vi "Element to JSON.vi"(8 "error in (no error)":errorcluster, 10 "Element":refnum<class "Config Element.lvclass">, 11 "Config-JSON":refnum<class "Config-JSON.lvclass">) -> (0 "error out":errorcluster, 2 "JSON":string)   [LabVIEW 2020, in "CDM-Config.lvlib" / "Config-JSON.lvclass"]
uses:
  Config-JSON.lvclass
  Config Element/Config Element.lvclass
  C:/dev/lv20CE/relink/lv-cdm/CDM-Config/Config Storage/Config Storage.lvclass
  Config Storage/Config Storage.lvclass
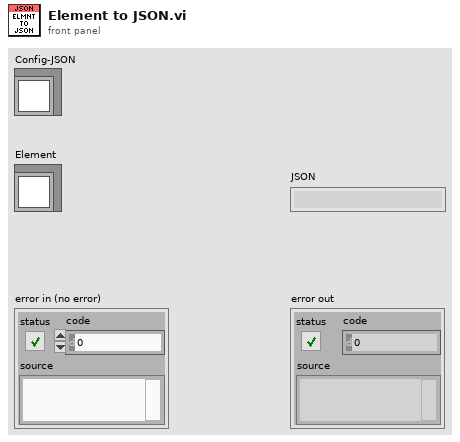
[diagram p1: front panel]
types:
  T1 = typedef "CDM-Config.lvlib/Value Type.ctl" = enum16{"String", "Number", "Bool", "Object", "Array"}
  T2 = typedef "CDM-Config.lvlib/Meta Data.ctl" = cluster{"Name":string, "Value":string}
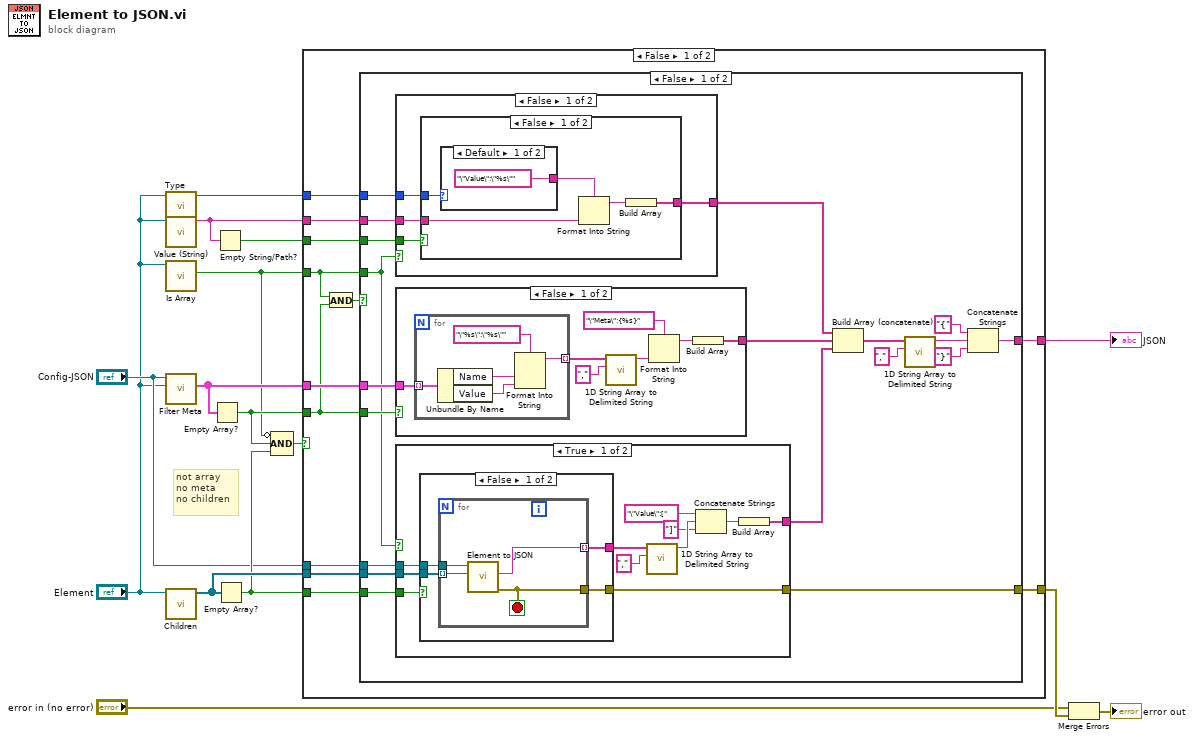
[diagram p0: block diagram]
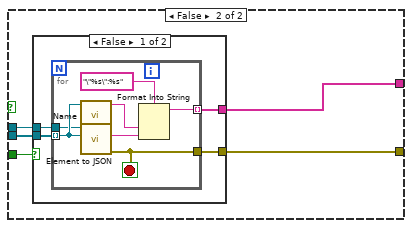
[diagram p3: hidden frame]
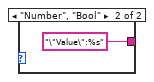
[diagram p5: hidden frame]
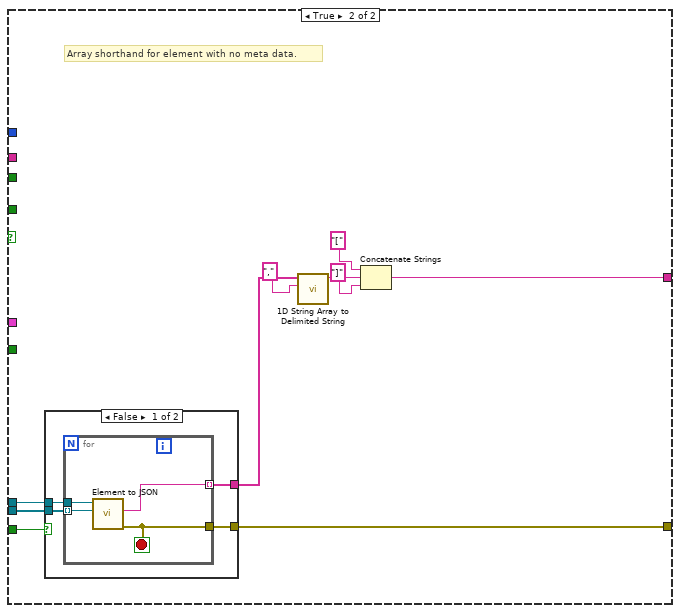
[diagram p9: hidden frame]
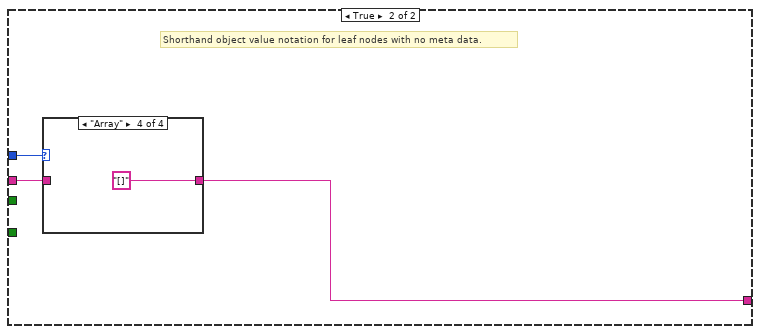
[diagram p11: hidden frame]
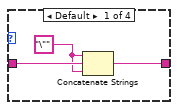
[diagram p12: hidden frame]
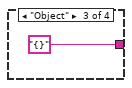
[diagram p14: hidden frame]
diagram:
  # "not array\nno meta\nno children"
  n1 = call "Type.vi"("Config Element in"="Element") -> ("Value Type"=w1:T1)  [unwired: 9 in, 1 out]
  n2 = call "Value (String).vi"("Config Element in"="Element") -> ("String Value"=w10:string)  [unwired: 9 in, 1 out]
  n3 = call "Is Array.vi"("Config Element in"="Element") -> ("Array"=w3:bool)  [unwired: 8 in, 2 out]
  n4 = call "Filter Meta.vi"("Element"="Element", "Config Storage in"="Config-JSON") -> ("Filtered Meta"=w5:T2[])  [unwired: 7 in, 2 out]
  n5 = call "Children.vi"("Config Element in"="Element") -> ("Elements"=w15:refnum<class "Config Element.lvclass">[])  [unwired: 9 in, 1 out]
  n6 = Empty Array?(array=w5) -> (empty?=w7:bool)
  n7 = Empty String/Path?(string/path=w10) -> (empty?=w9:bool)
  n8 = Empty Array?(array=w15) -> (empty?=w8:bool)
  n9 = Compound Arithmetic op=AND(invert w3, w7, w8) -> (w6:bool)
  n10 = case shown="False" w6 {
    tunnel: w15 -> [w27 _]
    tunnel: [w26 w123] -> w14
    tunnel: [w25 _] -> w13
    tunnel: w5 -> [w24 _]
    tunnel: w10 -> [w23 w124]
    tunnel: w9 -> [w22 _]
    tunnel: w8 -> [w21 _]
    tunnel: w7 -> [w19 _]
    tunnel: "Config-JSON" -> [w20 _]
    tunnel: w3 -> [w17 _]
    tunnel: w1 -> [w16 w125]
    frame False {
      n11 = And(x=w17, y=w19) -> (x .and. y?=w18:bool)
      n12 = case shown="False" w18 {
        tunnel: w27 -> [w46 w113]
        tunnel: [w40 w107] -> w26
        tunnel: [w39 w105] -> w25
        tunnel: w24 -> [w37 _]
        tunnel: w23 -> [w36 _]
        tunnel: w22 -> [w34 _]
        tunnel: w21 -> [w33 w112]
        tunnel: w20 -> [w32 w114]
        tunnel: w19 -> [w31 _]
        tunnel: w17 -> [w30 _]
        tunnel: w16 -> [w28 _]
        frame False {
          n13 = case shown="False" w30 {
            tunnel: w36 -> [w85 _]
            tunnel: [w84 _] -> w35
            tunnel: w34 -> [w83 _]
            tunnel: w28 -> [w82 _]
            frame False {
              n14 = case shown="False" w83 {
                tunnel: w85 -> [w88 _]
                tunnel: [w87 _] -> w84
                tunnel: w82 -> [w86 _]
                frame False {
                  n15 = case shown="Default" w86 {
                    tunnel: ["\"Value\":\"%s\"" ("format string") "\"Value\":%s" ("format string")] -> w90
                    frame Default {
                    }
                    frame "Number", "Bool" {
                    }
                  }
                  n16 = Format Into String(format string=w90, w88) -> (resulting string=w89:string)  [unwired: 2 in, 1 out]
                  n17 = Build Array(w89) -> (w87:string[])
                }
                frame True {
                }
              }
            }
            frame True {
            }
          }
          n18 = case shown="False" w31 {
            tunnel: [w93 _] -> w38
            tunnel: w37 -> [w94 _]
            frame False {
              n19 = for {
                tunnel: w94 -> [w104] mode=indexing
                tunnel: [w100] -> w98 mode=indexing
                n20 = Unbundle By Name(w104) -> ("Name"=w102:string, "Value"=w101:string)
                n21 = Format Into String(format string="\"%s\":\"%s\"", w102, w101) -> (resulting string=w100:string)  [unwired: 2 in, 1 out]
              }
              n22 = call <vilib>:"1D String Array to Delimited String.vi"("delimiter"=",", "string array"=w98) -> ("delimited string"=w96:string)  [unwired: 9 in]
              n23 = Format Into String(format string="\"Meta\":{%s}", w96) -> (resulting string=w95:string)  [unwired: 2 in, 1 out]
              n24 = Build Array(w95) -> (w93:string[])
            }
            frame True {
            }
          }
          n25 = case shown="True" w30 {
            tunnel: w46 -> [w57 w70]
            tunnel: [w56 w69] -> w39
            tunnel: w33 -> [w55 w68]
            tunnel: w32 -> [w54 w67]
            tunnel: [w47 w66] -> w29
            frame True {
              n26 = case shown="False" w55 {
                tunnel: w57 -> [w61 _]
                tunnel: [w59 _] -> w52
                tunnel: [w60 _] -> w56
                tunnel: w54 -> [w58 _]
                frame False {
                  n27 = for {
                    tunnel: w61 -> [w64] mode=indexing
                    tunnel: [w65] -> w60
                    tunnel: [w62] -> w59 mode=indexing
                    tunnel: w58 -> [w63]
                    stop <- w65 stop-if-true
                    n28 = call "Element to JSON.vi"("Element"=w64, "Config-JSON"=w63) -> ("error out"=w65:errorcluster, "JSON"=w62:string)  [unwired: 8 in]
                  }
                }
                frame True {
                }
              }
              n29 = call <vilib>:"1D String Array to Delimited String.vi"("delimiter"=",", "string array"=w52) -> ("delimited string"=w50:string)  [unwired: 9 in]
              n30 = Concatenate Strings("\"Value\":[", w50, "]" ("string")) -> (w48:string)
              n31 = Build Array(w48) -> (w47:string[])
            }
            frame False {
              n32 = case shown="False" w68 {
                tunnel: w70 -> [w74 _]
                tunnel: [w72 _] -> w66
                tunnel: [w73 _] -> w69
                tunnel: w67 -> [w71 _]
                frame False {
                  n33 = for {
                    tunnel: w74 -> [w80] mode=indexing
                    tunnel: [w81] -> w73
                    tunnel: [w76] -> w72 mode=indexing
                    tunnel: w71 -> [w75]
                    stop <- w81 stop-if-true
                    n34 = call "Name.vi"("Config Element in"=w80) -> ("Name"=w77:string)  [unwired: 9 in, 1 out]
                    n35 = call "Element to JSON.vi"("Element"=w80, "Config-JSON"=w75) -> ("error out"=w81:errorcluster, "JSON"=w78:string)  [unwired: 8 in]
                    n36 = Format Into String(format string="\"%s\":%s", w77, w78) -> (resulting string=w76:string)  [unwired: 2 in, 1 out]
                  }
                }
                frame True {
                }
              }
            }
          }
          n37 = Build Array (concatenate)(w35, w38, w29) -> (w44:string[])
          n38 = call <vilib>:"1D String Array to Delimited String.vi"("delimiter"=",", "string array"=w44) -> ("delimited string"=w43:string)  [unwired: 9 in]
          n39 = Concatenate Strings("{" ("string"), w43, "}" ("string")) -> (w40:string)
        }
        frame True {
          # "Array shorthand for element with no meta data."
          n40 = case shown="False" w112 {
            tunnel: w113 -> [w118 _]
            tunnel: [w116 _] -> w106
            tunnel: [w117 _] -> w105
            tunnel: w114 -> [w115 _]
            frame False {
              n41 = for {
                tunnel: w118 -> [w121] mode=indexing
                tunnel: [w122] -> w117
                tunnel: [w119] -> w116 mode=indexing
                tunnel: w115 -> [w120]
                stop <- w122 stop-if-true
                n42 = call "Element to JSON.vi"("Element"=w121, "Config-JSON"=w120) -> ("error out"=w122:errorcluster, "JSON"=w119:string)  [unwired: 8 in]
              }
            }
            frame True {
            }
          }
          n43 = call <vilib>:"1D String Array to Delimited String.vi"("delimiter"=",", "string array"=w106) -> ("delimited string"=w111:string)  [unwired: 9 in]
          n44 = Concatenate Strings("[" ("string"), w111, "]" ("string")) -> (w107:string)
        }
      }
    }
    frame True {
      # "Shorthand object value notation for leaf nodes with no meta data."
      n45 = case shown="\"Array\"" w125 {
        tunnel: w124 -> [w128 w129 _ _]
        tunnel: [w126 w129 "{}" ("String Value") "[]" ("String Value")] -> w123
        frame Default {
          w127 = "\""
          n46 = Concatenate Strings(w127, w128, w127) -> (w126:string)
        }
        frame "Number", "Bool" {
        }
        frame "Object" {
        }
        frame "Array" {
        }
      }
    }
  }
  "JSON" <- w14
  n47 = Merge Errors("error in (no error)", w13) -> (→"error out":errorcluster)
